vi "TpUnhandledMessage.vi"() -> (1 "tracepoint name":string)   [LabVIEW 2017, in "TraceLogger.lvlib"]
uses:
  <vilib>/addons/TraceLogger/TraceLogger.lvlib
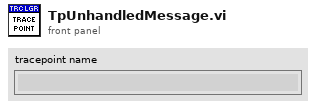
[diagram p1: front panel]
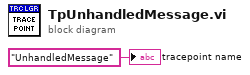
[diagram p0: block diagram]
diagram:
  "tracepoint name" <- "UnhandledMessage" ("ProcessName")
